vi "is a.vi"(8 "error in (no error)":errorcluster, 11 "Displacement Sensor in":refnum<class "DispSnsr.lvclass">) -> (0 "error out":errorcluster, 2 "is a":string, 3 "Displacement Sensor out":refnum<class "DispSnsr.lvclass">)   [LabVIEW 2016, in "Hardware.lvlib" / "Displacement Sensor.lvlib" / "DispSnsr.lvclass"]
uses:
  <userlib>/Common Components/Hardware/Displacement Sensor/DispSnsr/DispSnsr.lvclass
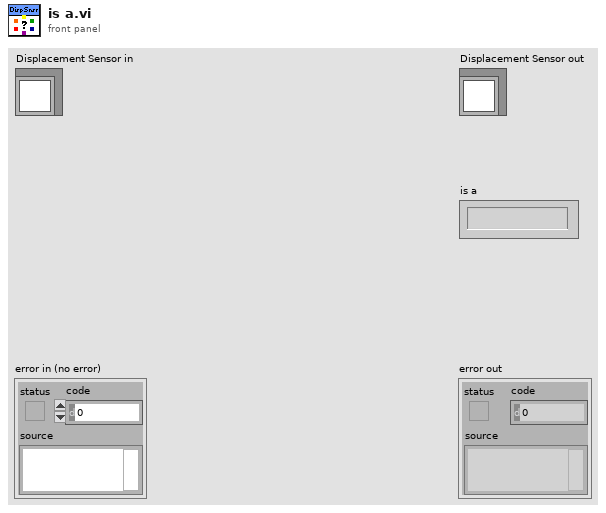
[diagram p1: front panel]
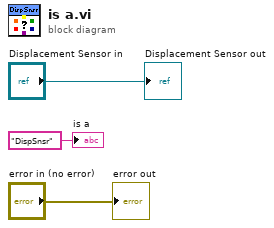
[diagram p0: block diagram]
diagram:
  "error out" <- "error in (no error)"
  "Displacement Sensor out" <- "Displacement Sensor in"
  "is a" <- "DispSnsr" ("is a")
